vi "TEST - Append or Replace Array Element.vi"(8 "error in (no error)":errorcluster) -> (0 "error out":errorcluster, 2 "Pass?":bool=TRUE)   [LabVIEW 2009]
doc: "This VI template can be used for the functional testing of VIs; this implementation includes handling for the testing of polymorphic VIs, and the polymorphic elements should be removed if not needed.\n\nCoded by Douglas A. Femec, January 24, 2006.\n\nCopyright (c) 2005-2006 MKS Instruments, Inc.\nAll rights reserved."
uses:
  TEST - Append or Replace Array Element - Inputs.ctl
  tests/Polymorphizer+ Data Type.ctl
  TEST - Append or Replace Array Element - Outputs.ctl
  Append or Replace Array Element/Append or Replace 1D Array Element (EXT).vi
  Append or Replace Array Element/Append or Replace 2D Array Element (EXT).vi
  Append or Replace Array Element/Append or Replace 1D Array Element (U64).vi
  Append or Replace Array Element/Append or Replace 2D Array Element (U64).vi
  Append or Replace Array Element/Append or Replace 1D Array Element (I64).vi
  Append or Replace Array Element/Append or Replace 2D Array Element (I64).vi
  Append or Replace Array Element/Append or Replace 1D Array Element (DBL).vi
  Append or Replace Array Element/Append or Replace 2D Array Element (DBL).vi
  Append or Replace Array Element/Append or Replace 1D Array Element (SGL).vi
  Append or Replace Array Element/Append or Replace 2D Array Element (SGL).vi
  Append or Replace Array Element/Append or Replace 1D Array Element (I32).vi
  Append or Replace Array Element/Append or Replace 2D Array Element (I32).vi
  Append or Replace Array Element/Append or Replace 1D Array Element (I16).vi
  Append or Replace Array Element/Append or Replace 2D Array Element (I16).vi
  Append or Replace Array Element/Append or Replace 1D Array Element (I8).vi
  Append or Replace Array Element/Append or Replace 2D Array Element (I8).vi
  Append or Replace Array Element/Append or Replace 1D Array Element (U32).vi
  Append or Replace Array Element/Append or Replace 2D Array Element (U32).vi
  Append or Replace Array Element/Append or Replace 1D Array Element (U16).vi
  Append or Replace Array Element/Append or Replace 2D Array Element (U16).vi
  Append or Replace Array Element/Append or Replace 1D Array Element (U8).vi
  Append or Replace Array Element/Append or Replace 2D Array Element (U8).vi
  Append or Replace Array Element/Append or Replace 1D Array Element (LVObject).vi
  Append or Replace Array Element/Append or Replace 2D Array Element (LVObject).vi
  Append or Replace Array Element/Append or Replace 1D Array Element (CXT).vi
  Append or Replace Array Element/Append or Replace 2D Array Element (CXT).vi
  Append or Replace Array Element/Append or Replace 1D Array Element (CDB).vi
  Append or Replace Array Element/Append or Replace 2D Array Element (CDB).vi
  Append or Replace Array Element/Append or Replace 1D Array Element (CSG).vi
  Append or Replace Array Element/Append or Replace 2D Array Element (CSG).vi
  Append or Replace Array Element/Append or Replace 1D Array Element (Boolean).vi
  Append or Replace Array Element/Append or Replace 2D Array Element (Boolean).vi
  Append or Replace Array Element/Append or Replace 1D Array Element (String).vi
  Append or Replace Array Element/Append or Replace 2D Array Element (String).vi
  Append or Replace Array Element/Append or Replace 1D Array Element (Path).vi
  Append or Replace Array Element/Append or Replace 2D Array Element (Path).vi
  Append or Replace Array Element/Append or Replace 1D Array Element (Variant).vi
  Append or Replace Array Element/Append or Replace 2D Array Element (Variant).vi
  tests/TestClass/TestClass.lvclass
panel:
  out "Generated Outputs":T1[][](array[typedef]) {"1D Array" format="%.2f"; "2D Array" format="%.2f"}
  in  "Expected Outputs":T1[](array[typedef])=[{"Description"="Expect 3 rows and 3 rows, 2 columns", "1D Array"=[0.0, 0.0, 1.0], "2D Array"=[[0.0, 0.0], [0.0, 0.0], [0.0, 1.0]]}, {"Description"="Expect 3 rows and 3 rows, 2 columns", "1D Array"=[1.0, 0.0, 1.0], "2D Array"=[[1.0, 0.0], [0.0, 1.0], [0.0, 1.0]]}, {"Description"="Expect 4 rows and 4 rows, 2 columns", "1D Array"=[0.0, 1.0, 1.0, 1.0], "2D Array"=[[0.0, 0.0], [1.0, 1.0], [0.0, 1.0], [1.0, 1.0]]}] {"1D Array" format="%.2f"; "2D Array" format="%.2f"}
  in  "Inputs":T2[](array[typedef])=[{"Row"=2, "Column"=1, "Description"="Append to empty array", "Data Types to Test"=[enum."EXT", enum."DBL", enum."SGL", enum."I32", enum."I16", enum."I8", enum."U32", enum."U16", enum."U8", enum."CXT", enum."CDB", enum."CSG", enum."Boolean", enum."String", enum."Path", enum."Variant", enum."I64", enum."U64", enum."LabVIEW Object"], "1D Array"=[], "2D Array"=[], "Element"=1.0}, {"Row"=2, "Column"=1, "Description"="Append to nearly filled array", "Data Types to Test"=[enum."EXT", enum."DBL", enum."SGL", enum."I32", enum."I16", enum."I8", enum."U32", enum."U16", enum."U8", enum."CXT", enum."CDB", enum."CSG", enum."Boolean", enum."String", enum."Path", enum."Variant", enum."I64", enum."U64", enum."LabVIEW Object"], "1D Array"=[1.0, 0.0], "2D Array"=[[1.0, 0.0], [0.0, 1.0]], "Element"=1.0}, {"Row"=2, "Column"=1, "Description"="Replace", "Data Types to Test"=[enum."EXT", enum."DBL", enum."SGL", enum."I32", enum."I16", enum."I8", enum."U32", enum."U16", enum."U8", enum."CXT", enum."CDB", enum."CSG", enum."Boolean", enum."String", enum."Path", enum."Variant", enum."I64", enum."U64", enum."LabVIEW Object"], "1D Array"=[0.0, 1.0, 0.0, 1.0], "2D Array"=[[0.0, 0.0], [1.0, 1.0], [0.0, 0.0], [1.0, 1.0]], "Element"=1.0}] {"Element" format="%.2f"; "1D Array" format="%.2f"; "2D Array" format="%.2f"}
  # "Copyright (c) 2005-2006 MKS Instruments, Inc.\nAll rights reserved."
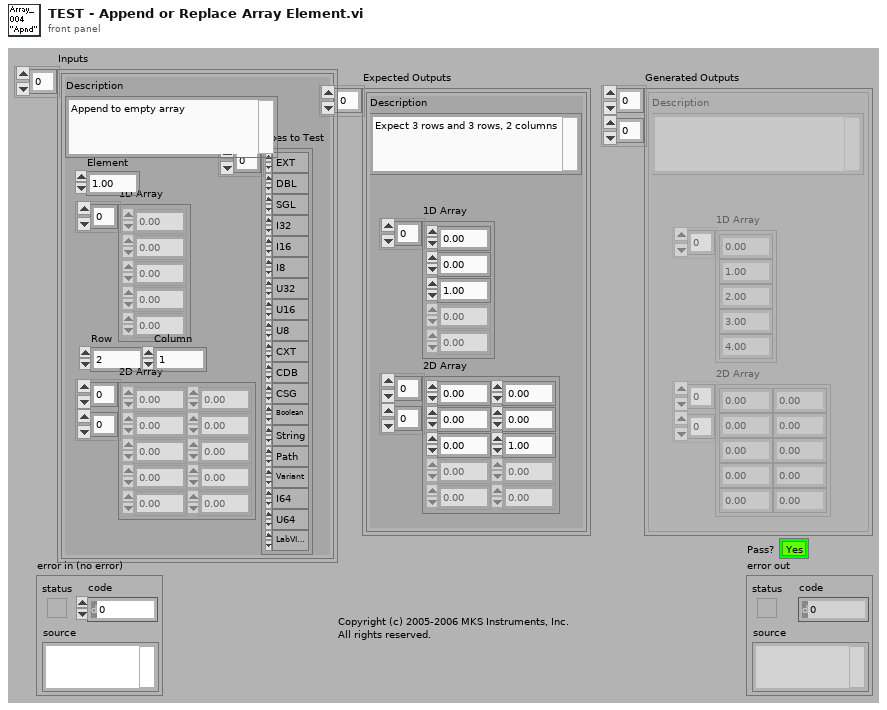
[diagram p1: front panel]
types:
  T1 = typedef "TEST - Append or Replace Array Element - Outputs.ctl" = cluster{"Description":string, "1D Array":sgl[], "2D Array":sgl[][]}
  T2 = typedef "TEST - Append or Replace Array Element - Inputs.ctl" = cluster{"Row":i32, "Column":i32, "Description":string, "Data Types to Test":T3[], "1D Array":sgl[], "2D Array":sgl[][], "Element":sgl}
  T3 = typedef "Polymorphizer+ Data Type.ctl" = enum16{"EXT", "DBL", "SGL", "I32", "I16", "I8", "U32", "U16", "U8", "CXT", "CDB", "CSG", "Boolean", "String", "Path", "Variant", "CTL-REF", "GEN-REF", "GObj-REF", "VI-REF", "ENUM", "ERR", "FILE-REF", "MENU-REF", "MENU-RING", "PICT-RING", "TXT&PICT-RING", "TXT-RING", "I64", "U64", "LabVIEW Object"}
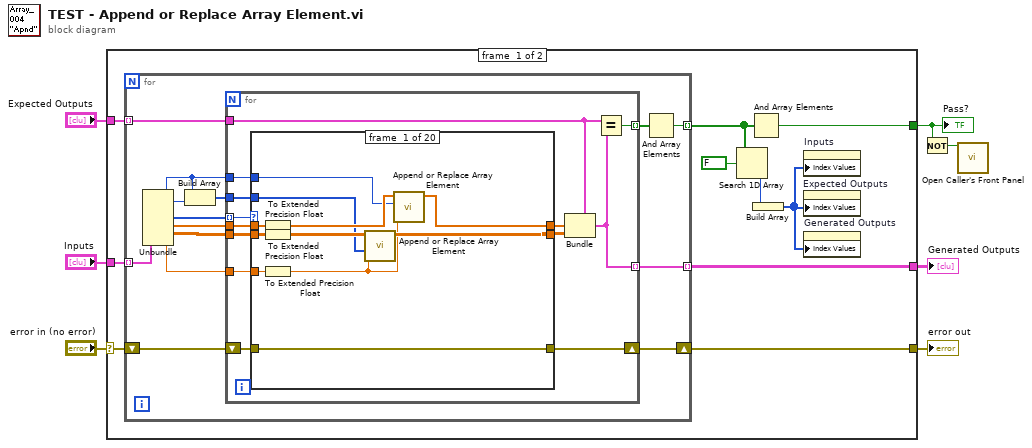
[diagram p0: block diagram]
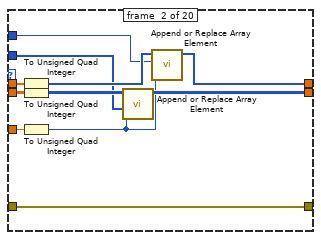
[diagram p2: hidden frame]
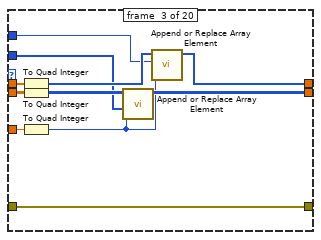
[diagram p3: hidden frame]
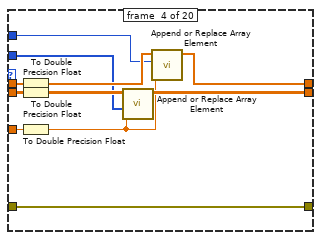
[diagram p4: hidden frame]
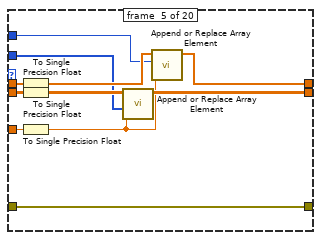
[diagram p5: hidden frame]
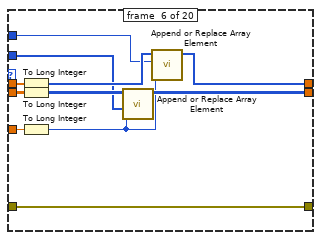
[diagram p6: hidden frame]
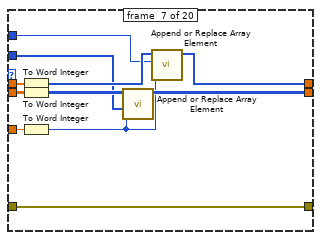
[diagram p7: hidden frame]
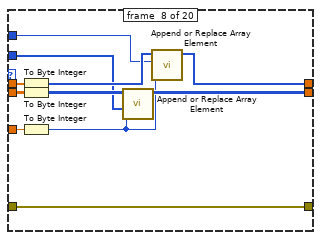
[diagram p8: hidden frame]
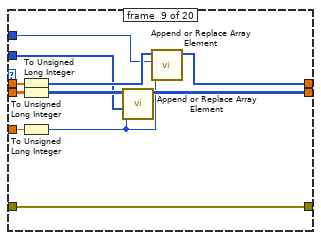
[diagram p9: hidden frame]
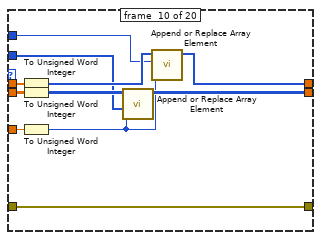
[diagram p10: hidden frame]
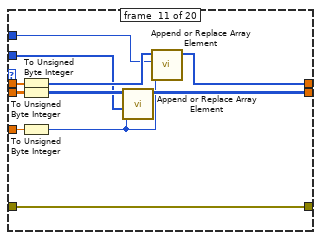
[diagram p11: hidden frame]
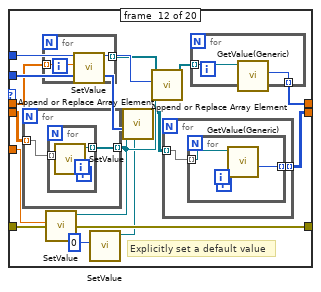
[diagram p12: hidden frame]
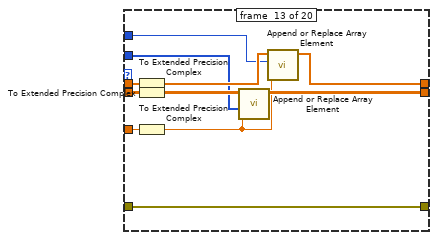
[diagram p13: hidden frame]
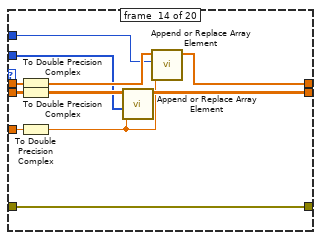
[diagram p14: hidden frame]
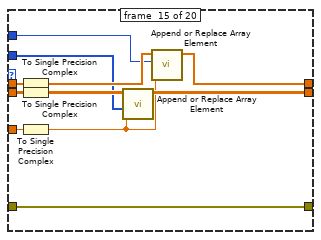
[diagram p15: hidden frame]
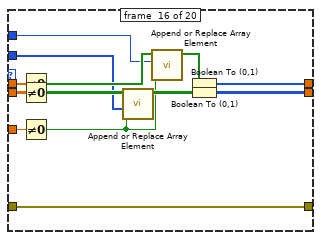
[diagram p16: hidden frame]
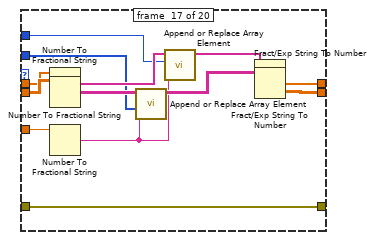
[diagram p17: hidden frame]
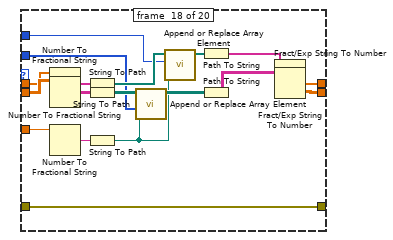
[diagram p18: hidden frame]
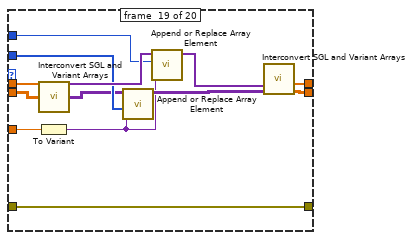
[diagram p19: hidden frame]
diagram:
  n1 = case shown="No Error" "error in (no error)" {
    selector: "error in (no error)" -> [w16 w286]
    tunnel: [w17 w286] -> w6
    tunnel: "Expected Outputs" -> [w14 _]
    tunnel: "Inputs" -> [w15 _]
    tunnel: [w13 _] -> w3
    tunnel: [w12 _] -> w1
    frame #0 {
      n2 = for {
        shift-right: [w26] -> w17
        shift-left: w16 -> [w27]
        tunnel: w15 -> [w28] mode=indexing
        tunnel: w14 -> [w31] mode=indexing
        tunnel: [w30] -> w13 mode=indexing
        tunnel: [w25] -> w11 mode=indexing
        n3 = Unbundle(w28) -> ("Row"=w19:i32, "Column"=w20:i32, "Data Types to Test"=w24:T3[], "1D Array"=w23:sgl[], "2D Array"=w22:sgl[][], "Element"=w21:sgl)  [unwired: 1 out]
        n4 = Build Array(w19, w20) -> (w18:i32[])
        n5 = for {
          tunnel: w31 -> [w44]
          tunnel: [w42] -> w30 mode=indexing
          tunnel: [w43] -> w29 mode=indexing
          shift-right: [w37] -> w26
          shift-left: w27 -> [w38]
          tunnel: w24 -> [w39] mode=indexing
          tunnel: w23 -> [w41]
          tunnel: w22 -> [w40]
          tunnel: w21 -> [w34]
          tunnel: w19 -> [w33]
          tunnel: w18 -> [w32]
          n6 = case shown="\"LabVIEW Object\"" w39 {
            tunnel: w41 -> [w54 w65 w76 w87 w98 w109 w120 w131 w142 w153 w164 w177 w202 w213 w224 w237 w250 w266 w280 w284]
            tunnel: [w51 w62 w73 w84 w95 w106 w117 w128 w139 w150 w161 w168 w199 w210 w221 w227 w242 w259 w272 w284] -> w36
            tunnel: [w50 w61 w72 w83 w94 w105 w116 w127 w138 w149 w160 w170 w198 w209 w220 w228 w241 w260 w274 w283] -> w35
            tunnel: w40 -> [w55 w66 w77 w88 w99 w110 w121 w132 w143 w154 w165 w173 w203 w214 w225 w238 w251 w268 w281 w283]
            tunnel: w38 -> [w52 w63 w74 w85 w96 w107 w118 w129 w140 w151 w162 w180 w200 w211 w222 w235 w249 w265 w282 w285]
            tunnel: [w52 w63 w74 w85 w96 w107 w118 w129 w140 w151 w162 w180 w200 w211 w222 w235 w249 w265 w282 w285] -> w37
            tunnel: w34 -> [w48 w59 w70 w81 w92 w103 w114 w125 w136 w147 w158 w175 w196 w207 w218 w231 w240 w255 w271 _]
            tunnel: w33 -> [w47 w58 w69 w80 w91 w102 w113 w124 w135 w146 w157 w179 w195 w206 w217 w230 w245 w258 w277 _]
            tunnel: w32 -> [w46 w57 w68 w79 w90 w101 w112 w123 w134 w145 w156 w178 w194 w205 w216 w229 w246 w257 w278 _]
            frame #0 {
              n7 = To Extended Precision Float(1:w54) -> (0:w53:ext[])
              n8 = To Extended Precision Float(1:w55) -> (0:w49:ext[][])
              n9 = To Extended Precision Float(1:w48) -> (0:w45:ext)
              n10 = call-poly "Append or Replace Array Element.vi"("Element"=w45, "Indices (>=1D)"=w46, "Array In"=w49) -> ("Array Out"=w50:ext[][])  [unwired: 8 in]
              n11 = call-poly "Append or Replace Array Element.vi"("Element"=w45, "Index (1D)"=w47, "Array In"=w53) -> ("Array Out"=w51:ext[])  [unwired: 8 in]
            }
            frame #1 {
              n12 = To Unsigned Quad Integer(1:w65) -> (0:w64:u64[])
              n13 = To Unsigned Quad Integer(1:w66) -> (0:w60:u64[][])
              n14 = To Unsigned Quad Integer(1:w59) -> (0:w56:u64)
              n15 = call-poly "Append or Replace Array Element.vi"("Element"=w56, "Indices (>=1D)"=w57, "Array In"=w60) -> ("Array Out"=w61:u64[][])  [unwired: 8 in]
              n16 = call-poly "Append or Replace Array Element.vi"("Element"=w56, "Index (1D)"=w58, "Array In"=w64) -> ("Array Out"=w62:u64[])  [unwired: 8 in]
            }
            frame #2 {
              n17 = To Quad Integer(1:w76) -> (0:w75:i64[])
              n18 = To Quad Integer(1:w77) -> (0:w71:i64[][])
              n19 = To Quad Integer(1:w70) -> (0:w67:i64)
              n20 = call-poly "Append or Replace Array Element.vi"("Element"=w67, "Indices (>=1D)"=w68, "Array In"=w71) -> ("Array Out"=w72:i64[][])  [unwired: 8 in]
              n21 = call-poly "Append or Replace Array Element.vi"("Element"=w67, "Index (1D)"=w69, "Array In"=w75) -> ("Array Out"=w73:i64[])  [unwired: 8 in]
            }
            frame #3 {
              n22 = To Double Precision Float(number=w87) -> (double precision float=w86:dbl[])
              n23 = To Double Precision Float(number=w88) -> (double precision float=w82:dbl[][])
              n24 = To Double Precision Float(number=w81) -> (double precision float=w78:dbl)
              n25 = call-poly "Append or Replace Array Element.vi"("Element"=w78, "Indices (>=1D)"=w79, "Array In"=w82) -> ("Array Out"=w83:dbl[][])  [unwired: 8 in]
              n26 = call-poly "Append or Replace Array Element.vi"("Element"=w78, "Index (1D)"=w80, "Array In"=w86) -> ("Array Out"=w84:dbl[])  [unwired: 8 in]
            }
            frame #4 {
              n27 = To Single Precision Float(number=w98) -> (single precision float=w97:sgl[])
              n28 = To Single Precision Float(number=w99) -> (single precision float=w93:sgl[][])
              n29 = To Single Precision Float(number=w92) -> (single precision float=w89:sgl)
              n30 = call-poly "Append or Replace Array Element.vi"("Element"=w89, "Indices (>=1D)"=w90, "Array In"=w93) -> ("Array Out"=w94:sgl[][])  [unwired: 8 in]
              n31 = call-poly "Append or Replace Array Element.vi"("Element"=w89, "Index (1D)"=w91, "Array In"=w97) -> ("Array Out"=w95:sgl[])  [unwired: 8 in]
            }
            frame #5 {
              n32 = To Long Integer(number=w109) -> (32bit integer=w108:i32[])
              n33 = To Long Integer(number=w110) -> (32bit integer=w104:i32[][])
              n34 = To Long Integer(number=w103) -> (32bit integer=w100:i32)
              n35 = call-poly "Append or Replace Array Element.vi"("Element"=w100, "Indices (>=1D)"=w101, "Array In"=w104) -> ("Array Out"=w105:i32[][])  [unwired: 8 in]
              n36 = call-poly "Append or Replace Array Element.vi"("Element"=w100, "Index (1D)"=w102, "Array In"=w108) -> ("Array Out"=w106:i32[])  [unwired: 8 in]
            }
            frame #6 {
              n37 = To Word Integer(number=w120) -> (16bit integer=w119:i16[])
              n38 = To Word Integer(number=w121) -> (16bit integer=w115:i16[][])
              n39 = To Word Integer(number=w114) -> (16bit integer=w111:i16)
              n40 = call-poly "Append or Replace Array Element.vi"("Element"=w111, "Indices (>=1D)"=w112, "Array In"=w115) -> ("Array Out"=w116:i16[][])  [unwired: 8 in]
              n41 = call-poly "Append or Replace Array Element.vi"("Element"=w111, "Index (1D)"=w113, "Array In"=w119) -> ("Array Out"=w117:i16[])  [unwired: 8 in]
            }
            frame #7 {
              n42 = To Byte Integer(number=w131) -> (8bit integer=w130:i8[])
              n43 = To Byte Integer(number=w132) -> (8bit integer=w126:i8[][])
              n44 = To Byte Integer(number=w125) -> (8bit integer=w122:i8)
              n45 = call-poly "Append or Replace Array Element.vi"("Element"=w122, "Indices (>=1D)"=w123, "Array In"=w126) -> ("Array Out"=w127:i8[][])  [unwired: 8 in]
              n46 = call-poly "Append or Replace Array Element.vi"("Element"=w122, "Index (1D)"=w124, "Array In"=w130) -> ("Array Out"=w128:i8[])  [unwired: 8 in]
            }
            frame #8 {
              n47 = To Unsigned Long Integer(number=w142) -> (unsigned 32bit integer=w141:u32[])
              n48 = To Unsigned Long Integer(number=w143) -> (unsigned 32bit integer=w137:u32[][])
              n49 = To Unsigned Long Integer(number=w136) -> (unsigned 32bit integer=w133:u32)
              n50 = call-poly "Append or Replace Array Element.vi"("Element"=w133, "Indices (>=1D)"=w134, "Array In"=w137) -> ("Array Out"=w138:u32[][])  [unwired: 8 in]
              n51 = call-poly "Append or Replace Array Element.vi"("Element"=w133, "Index (1D)"=w135, "Array In"=w141) -> ("Array Out"=w139:u32[])  [unwired: 8 in]
            }
            frame #9 {
              n52 = To Unsigned Word Integer(number=w153) -> (unsigned 16bit integer=w152:u16[])
              n53 = To Unsigned Word Integer(number=w154) -> (unsigned 16bit integer=w148:u16[][])
              n54 = To Unsigned Word Integer(number=w147) -> (unsigned 16bit integer=w144:u16)
              n55 = call-poly "Append or Replace Array Element.vi"("Element"=w144, "Indices (>=1D)"=w145, "Array In"=w148) -> ("Array Out"=w149:u16[][])  [unwired: 8 in]
              n56 = call-poly "Append or Replace Array Element.vi"("Element"=w144, "Index (1D)"=w146, "Array In"=w152) -> ("Array Out"=w150:u16[])  [unwired: 8 in]
            }
            frame #10 {
              n57 = To Unsigned Byte Integer(number=w164) -> (unsigned 8bit integer=w163:u8[])
              n58 = To Unsigned Byte Integer(number=w165) -> (unsigned 8bit integer=w159:u8[][])
              n59 = To Unsigned Byte Integer(number=w158) -> (unsigned 8bit integer=w155:u8)
              n60 = call-poly "Append or Replace Array Element.vi"("Element"=w155, "Indices (>=1D)"=w156, "Array In"=w159) -> ("Array Out"=w160:u8[][])  [unwired: 8 in]
              n61 = call-poly "Append or Replace Array Element.vi"("Element"=w155, "Index (1D)"=w157, "Array In"=w163) -> ("Array Out"=w161:u8[])  [unwired: 8 in]
            }
            frame #11 {
              # "Explicitly set a default value"
              n62 = for {
                tunnel: [w188] -> w172 mode=indexing
                tunnel: w173 -> [w187] mode=indexing
                n63 = for {
                  tunnel: w187 -> [w190] mode=indexing
                  tunnel: [w189] -> w188 mode=indexing
                  n64 = call "SetValue.vi"("Value"=w190) -> ("TestClass out"=w189:refnum<class "TestClass.lvclass">)  [unwired: 9 in, 1 out]
                }
              }
              n65 = for {
                tunnel: w177 -> [w192] mode=indexing
                tunnel: [w191] -> w176 mode=indexing
                n66 = call "SetValue.vi"("Value"=w192) -> ("TestClass out"=w191:refnum<class "TestClass.lvclass">)  [unwired: 9 in, 1 out]
              }
              n67 = call "SetValue.vi"("Value"=w175) -> ("TestClass out"=w174:refnum<class "TestClass.lvclass">)  [unwired: 9 in, 1 out]
              n68 = call "SetValue.vi"("Value"=0) -> ("TestClass out"=w166:refnum<class "TestClass.lvclass">)  [unwired: 9 in, 1 out]
              n69 = call-poly "Append or Replace Array Element.vi"("Default"=w166, "Element"=w174, "Indices (>=1D)"=w178, "Array In"=w172) -> ("Array Out"=w171:refnum<class>[][])  [unwired: 7 in]
              n70 = call-poly "Append or Replace Array Element.vi"("Element"=w174, "Index (1D)"=w179, "Array In"=w176) -> ("Array Out"=w169:refnum<class>[])  [unwired: 8 in]
              n71 = for {
                tunnel: w171 -> [w184] mode=indexing
                tunnel: [w183] -> w170 mode=indexing
                n72 = for {
                  tunnel: w184 -> [w186] mode=indexing
                  tunnel: [w185] -> w183 mode=indexing
                  n73 = call "GetValue(Generic).vi"("TestClass in"=w186) -> ("Value"=w185:i32)  [unwired: 8 in, 2 out]
                }
              }
              n74 = for {
                tunnel: w169 -> [w182] mode=indexing
                tunnel: [w181] -> w168 mode=indexing
                n75 = call "GetValue(Generic).vi"("TestClass in"=w182) -> ("Value"=w181:i32)  [unwired: 8 in, 2 out]
              }
            }
            frame #12 {
              n76 = To Extended Precision Complex(1:w202) -> (0:w201:cxt[])
              n77 = To Extended Precision Complex(1:w203) -> (0:w197:cxt[][])
              n78 = To Extended Precision Complex(1:w196) -> (0:w193:cxt)
              n79 = call-poly "Append or Replace Array Element.vi"("Element"=w193, "Indices (>=1D)"=w194, "Array In"=w197) -> ("Array Out"=w198:cxt[][])  [unwired: 8 in]
              n80 = call-poly "Append or Replace Array Element.vi"("Element"=w193, "Index (1D)"=w195, "Array In"=w201) -> ("Array Out"=w199:cxt[])  [unwired: 8 in]
            }
            frame #13 {
              n81 = To Double Precision Complex(1:w213) -> (0:w212:cdb[])
              n82 = To Double Precision Complex(1:w214) -> (0:w208:cdb[][])
              n83 = To Double Precision Complex(1:w207) -> (0:w204:cdb)
              n84 = call-poly "Append or Replace Array Element.vi"("Element"=w204, "Indices (>=1D)"=w205, "Array In"=w208) -> ("Array Out"=w209:cdb[][])  [unwired: 8 in]
              n85 = call-poly "Append or Replace Array Element.vi"("Element"=w204, "Index (1D)"=w206, "Array In"=w212) -> ("Array Out"=w210:cdb[])  [unwired: 8 in]
            }
            frame #14 {
              n86 = To Single Precision Complex(1:w224) -> (0:w223:csg[])
              n87 = To Single Precision Complex(1:w225) -> (0:w219:csg[][])
              n88 = To Single Precision Complex(1:w218) -> (0:w215:csg)
              n89 = call-poly "Append or Replace Array Element.vi"("Element"=w215, "Indices (>=1D)"=w216, "Array In"=w219) -> ("Array Out"=w220:csg[][])  [unwired: 8 in]
              n90 = call-poly "Append or Replace Array Element.vi"("Element"=w215, "Index (1D)"=w217, "Array In"=w223) -> ("Array Out"=w221:csg[])  [unwired: 8 in]
            }
            frame #15 {
              n91 = Not Equal To 0?(x=w237) -> (x != 0?=w236:bool[])
              n92 = Not Equal To 0?(x=w238) -> (x != 0?=w232:bool[][])
              n93 = Not Equal To 0?(x=w231) -> (x != 0?=w226:bool)
              n94 = call-poly "Append or Replace Array Element.vi"("Element"=w226, "Indices (>=1D)"=w229, "Array In"=w232) -> ("Array Out"=w233:bool[][])  [unwired: 8 in]
              n95 = call-poly "Append or Replace Array Element.vi"("Element"=w226, "Index (1D)"=w230, "Array In"=w236) -> ("Array Out"=w234:bool[])  [unwired: 8 in]
              n96 = Boolean To (0,1)(Boolean=w234) -> (0, 1=w227:i16[])
              n97 = Boolean To (0,1)(Boolean=w233) -> (0, 1=w228:i16[][])
            }
            frame #16 {
              n98 = Number To Fractional String(number=w250) -> (F-format string=w248:string[])  [unwired: 3 in]
              n99 = Number To Fractional String(number=w251) -> (F-format string=w247:string[][])  [unwired: 3 in]
              n100 = Number To Fractional String(number=w240) -> (F-format string=w239:string)  [unwired: 3 in]
              n101 = call-poly "Append or Replace Array Element.vi"("Element"=w239, "Indices (>=1D)"=w246, "Array In"=w247) -> ("Array Out"=w243:string[][])  [unwired: 8 in]
              n102 = call-poly "Append or Replace Array Element.vi"("Element"=w239, "Index (1D)"=w245, "Array In"=w248) -> ("Array Out"=w244:string[])  [unwired: 8 in]
              n103 = Fract/Exp String To Number(string=w244) -> (number=w242:dbl[])  [unwired: 3 in, 1 out]
              n104 = Fract/Exp String To Number(string=w243) -> (number=w241:dbl[][])  [unwired: 3 in, 1 out]
            }
            frame #17 {
              n105 = Number To Fractional String(number=w266) -> (F-format string=w267:string[])  [unwired: 3 in]
              n106 = Number To Fractional String(number=w268) -> (F-format string=w269:string[][])  [unwired: 3 in]
              n107 = Number To Fractional String(number=w255) -> (F-format string=w256:string)  [unwired: 3 in]
              n108 = String To Path(string=w267) -> (path=w264:path[])
              n109 = String To Path(string=w269) -> (path=w261:path[][])
              n110 = String To Path(string=w256) -> (path=w252:path)
              n111 = call-poly "Append or Replace Array Element.vi"("Element"=w252, "Indices (>=1D)"=w257, "Array In"=w261) -> ("Array Out"=w262:path[][])  [unwired: 8 in]
              n112 = call-poly "Append or Replace Array Element.vi"("Element"=w252, "Index (1D)"=w258, "Array In"=w264) -> ("Array Out"=w263:path[])  [unwired: 8 in]
              n113 = Path To String(path=w263) -> (string=w254:string[])
              n114 = Path To String(path=w262) -> (string=w253:string[][])
              n115 = Fract/Exp String To Number(string=w254) -> (number=w259:dbl[])  [unwired: 3 in, 1 out]
              n116 = Fract/Exp String To Number(string=w253) -> (number=w260:dbl[][])  [unwired: 3 in, 1 out]
            }
            frame #18 {
              n117 = call "Interconvert SGL and Variant Arrays.vi"("SGL 1D Array In"=w280, "SGL 2D Array In"=w281) -> ("Variant 1D Array Out"=w279:variant[], "Variant 2D Array Out"=w275:variant[][])  [unwired: 9 in, 3 out]
              n118 = To Variant(anything=w271) -> (Variant=w270:variant)
              n119 = call-poly "Append or Replace Array Element.vi"("Element"=w270, "Indices (>=1D)"=w278, "Array In"=w275) -> ("Array Out"=w276:variant[][])  [unwired: 8 in]
              n120 = call-poly "Append or Replace Array Element.vi"("Element"=w270, "Index (1D)"=w277, "Array In"=w279) -> ("Array Out"=w273:variant[])  [unwired: 8 in]
              n121 = call "Interconvert SGL and Variant Arrays.vi"("Variant 1D Array In"=w273, "Variant 2D Array In"=w276) -> ("SGL 1D Array Out"=w272:sgl[], "SGL 2D Array Out"=w274:sgl[][])  [unwired: 9 in, 3 out]
            }
            frame #19 {
            }
          }
          n122 = Bundle(cluster=w44, "1D Array"=w36, "2D Array"=w35) -> (w42:T1)  [unwired: 1 in]
          n123 = Equal?(x=w44, y=w42) -> (x = y?=w43:bool)
        }
        n124 = And Array Elements(Boolean array=w29) -> (logical AND=w25:bool)
      }
      n125 = Search 1D Array(1D array=w11, element=FALSE) -> (index of element=w9:i32)  [unwired: 1 in]
      n126 = And Array Elements(Boolean array=w11) -> (logical AND=w12:bool)
      n127 = Build Array(w9) -> (w8:i32[])
      n128 = property on="Inputs" class="Arr (strict)"("Index Values"=w8) -> ()  [unwired: 2 in, 2 out]
      n129 = property on="Expected Outputs" class="Arr (strict)"("Index Values"=w8) -> ()  [unwired: 2 in, 2 out]
      n130 = property on="Generated Outputs" class="Arr (strict)"("Index Values"=w8) -> ()  [unwired: 2 in, 2 out]
    }
    frame #1 {
    }
  }
  "error out" <- w6
  "Pass?" <- w1
  "Generated Outputs" <- w3
  n131 = Not(x=w1) -> (.not. x?=w2:bool)
  n132 = call "Open Caller's Front Panel.vi"("Open?"=w2) -> ()  [unwired: 14 in, 1 out]
